vi "Get Port Widths in Bits.vi"(11 "niInstr AXI4-Stream Writer FXP64x1 v1 FPGA in":refnum<class "niInstr AXI4-Stream Writer FXP64x1 v1 FPGA.lvclass">) -> (2 "port widths":T1, 3 "niInstr AXI4-Stream Writer FXP64x1 v1 FPGA out":refnum<class "niInstr AXI4-Stream Writer FXP64x1 v1 FPGA.lvclass">)   [LabVIEW 2015, in "niInstr AXI4-Stream Writer FXP64x1 v1 FPGA.lvclass"]
uses:
  <instrlib>/_niInstr/CLIP Adapters/v1/FPGA/AXI4-Stream/Writer FXP64x1/niInstr AXI4-Stream Writer FXP64x1 v1 FPGA.lvclass
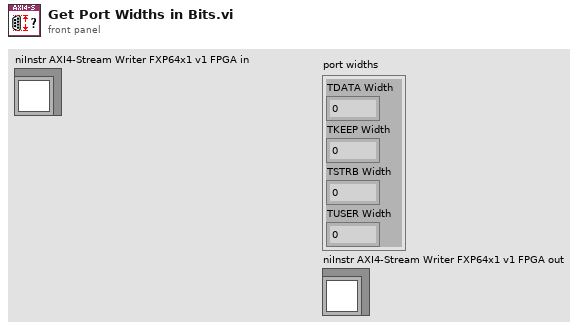
[diagram p1: front panel]
types:
  T1 = cluster{"TDATA Width":i16, "TKEEP Width":i16, "TSTRB Width":i16, "TUSER Width":i16}
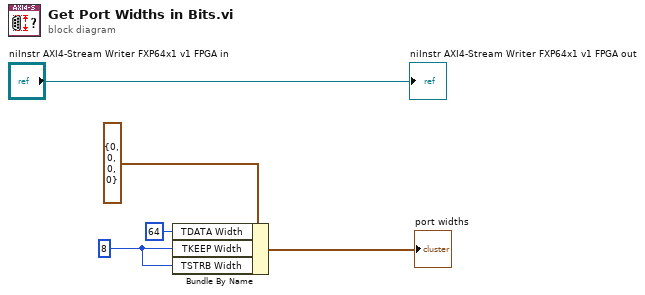
[diagram p0: block diagram]
diagram:
  w2 = i16 8 ("TDATA Width")
  n1 = Bundle By Name(cluster=T1 {"TDATA Width"=0, "TKEEP Width"=0, "TSTRB Width"=0, "TUSER Width"=0} ("Port Widths"), "TDATA Width"=i16 64, "TKEEP Width"=w2, "TSTRB Width"=w2) -> (→"port widths":T1)
  "niInstr AXI4-Stream Writer FXP64x1 v1 FPGA out" <- "niInstr AXI4-Stream Writer FXP64x1 v1 FPGA in"
